vi "Ejercicio 2.3.vi"() -> ()   [LabVIEW 2021]
uses:
  <vilib>/express/express arith-compare/Formula/XNode/ExpressFormulaBlockNode.xnode
panel:
  out "Numeric 3":dbl
  in  "Numeric":dbl
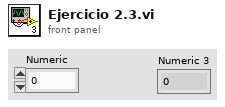
[diagram p1: front panel]
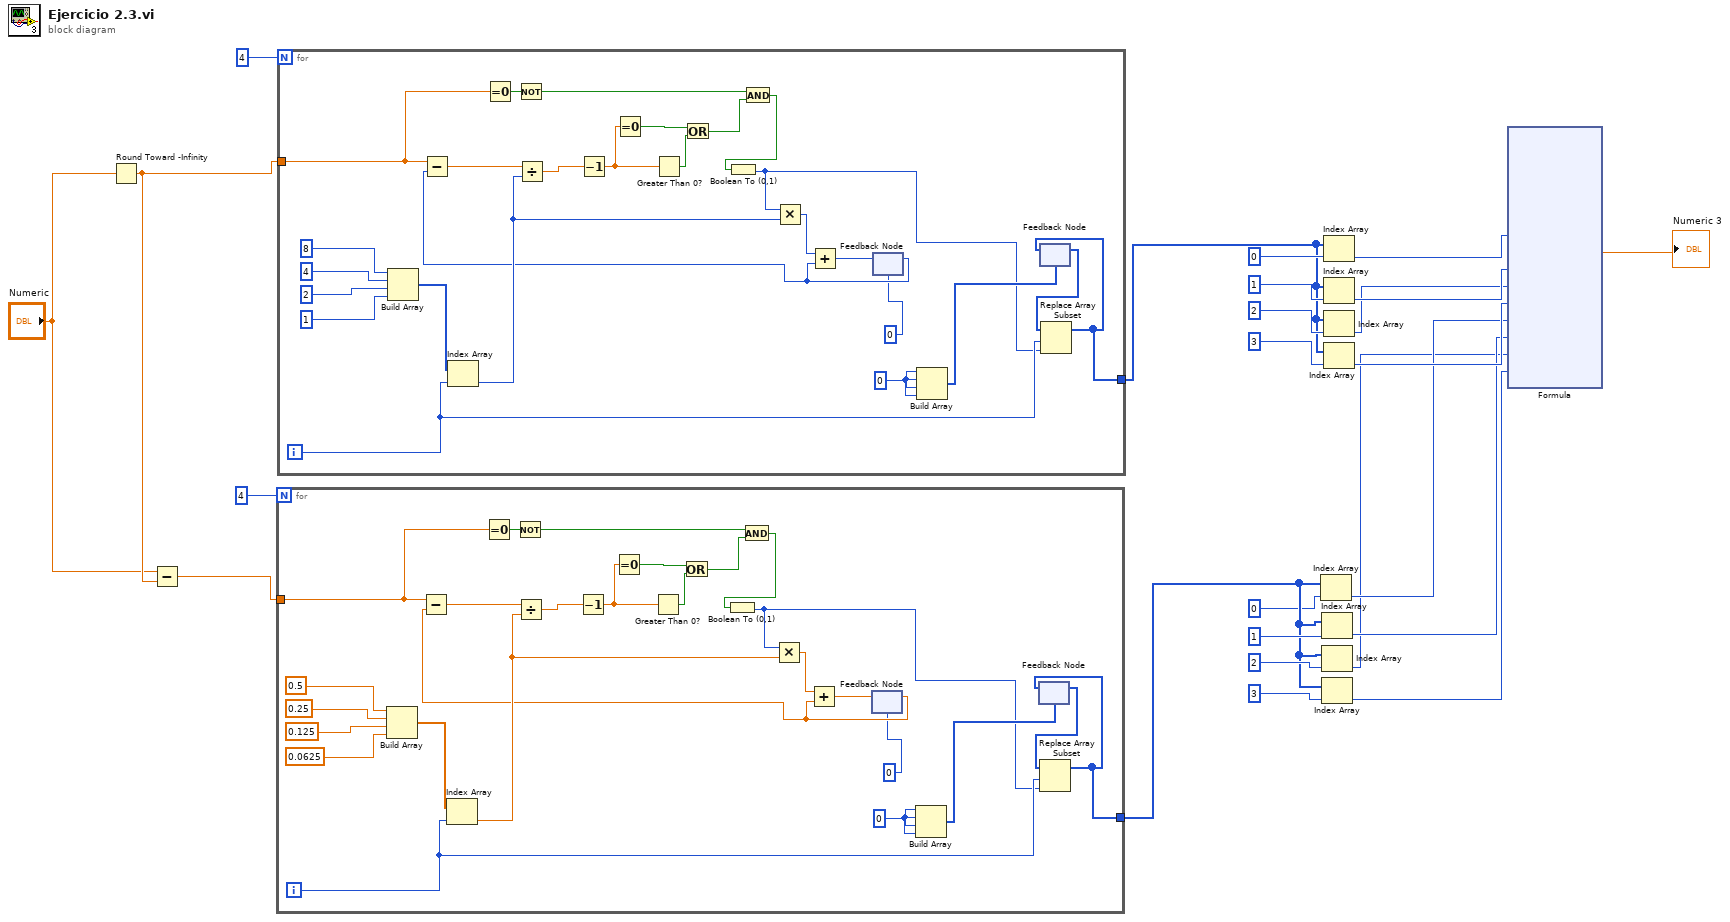
[diagram p0: block diagram]
diagram:
  n1 = Round Toward -Infinity(1:"Numeric") -> (0:w23:dbl)
  n2 = Subtract(x="Numeric", y=w23) -> (x-y=w3:dbl)
  n3 = for {
    N: 4 -> [_]
    tunnel: w3 -> [w43]
    tunnel: [w29] -> w2
    i -> [w34]
    w33 = 0
    n4 = Build Array(0.5, 0.25, 0.125, 0.0625) -> (w50:dbl[])
    n5 = Index Array(array=w50, index=w34) -> (element=w38:dbl)
    n6 = Equal To 0?(x=w43) -> (x = 0?=w45:bool)
    n7 = Not(x=w45) -> (.not. x?=w44:bool)
    n8 = feedback #1(0) -> (w36:dbl)
    n9 = Subtract(x=w43, y=w36) -> (x-y=w42:dbl)
    n10 = Divide(x=w42, y=w38) -> (x/y=w40:dbl)
    n11 = Decrement(x=w40) -> (x-1=w39:dbl)
    n12 = Equal To 0?(x=w39) -> (x = 0?=w49:bool)
    n13 = Greater Than 0?(x=w39) -> (x > 0?=w48:bool)
    n14 = Or(x=w49, y=w48) -> (x .or. y?=w46:bool)
    n15 = And(x=w44, y=w46) -> (x .and. y?=w41:bool)
    n16 = Boolean To (0,1)(Boolean=w41) -> (0, 1=w30:i16)
    n17 = Multiply(x=w30, y=w38) -> (x*y=w47:dbl)
    n18 = Add(x=w47, y=w36) -> (x+y=w37:dbl)
    n19 = feedback-in #1(w37) -> ()
    n20 = Build Array(w33, w33, w33, w33) -> (w31:i32[])
    n21 = feedback #2(w31) -> (w32:i32[])
    n22 = Replace Array Subset(array=w32, new element=w30, index=w34) -> (w29:i32[])
    n23 = feedback-in #2(w29) -> ()
  }
  n24 = for {
    N: 4 -> [_]
    tunnel: w23 -> [w65]
    tunnel: [w51] -> w17
    i -> [w56]
    w55 = 0
    n25 = Build Array(8, 4, 2, 1) -> (w72:i32[])
    n26 = Index Array(array=w72, index=w56) -> (element=w60:i32)
    n27 = Equal To 0?(x=w65) -> (x = 0?=w67:bool)
    n28 = Not(x=w67) -> (.not. x?=w66:bool)
    n29 = feedback #3(0) -> (w58:i32)
    n30 = Subtract(x=w65, y=w58) -> (x-y=w64:dbl)
    n31 = Divide(x=w64, y=w60) -> (x/y=w62:dbl)
    n32 = Decrement(x=w62) -> (x-1=w61:dbl)
    n33 = Equal To 0?(x=w61) -> (x = 0?=w71:bool)
    n34 = Greater Than 0?(x=w61) -> (x > 0?=w70:bool)
    n35 = Or(x=w71, y=w70) -> (x .or. y?=w68:bool)
    n36 = And(x=w66, y=w68) -> (x .and. y?=w63:bool)
    n37 = Boolean To (0,1)(Boolean=w63) -> (0, 1=w52:i16)
    n38 = Multiply(x=w52, y=w60) -> (x*y=w69:i32)
    n39 = Add(x=w69, y=w58) -> (x+y=w59:i32)
    n40 = feedback-in #3(w59) -> ()
    n41 = Build Array(w55, w55, w55, w55) -> (w53:i32[])
    n42 = feedback #4(w53) -> (w54:i32[])
    n43 = Replace Array Subset(array=w54, new element=w52, index=w56) -> (w51:i32[])
    n44 = feedback-in #4(w51) -> ()
  }
  n45 = Index Array(array=w2, index=0) -> (element=w9:i32)
  n46 = Index Array(array=w2, index=1) -> (element=w8:i32)
  n47 = Index Array(array=w2, index=2) -> (element=w5:i32)
  n48 = Index Array(array=w2, index=3) -> (element=w7:i32)
  n49 = Index Array(array=w17, index=0) -> (element=w11:i32)
  n50 = Index Array(array=w17, index=1) -> (element=w13:i32)
  n51 = Index Array(array=w17, index=2) -> (element=w12:i32)
  n52 = Index Array(array=w17, index=3) -> (element=w10:i32)
  n53 = xnode "Formula"("X1"=w11, "X2"=w13, "X3"=w12, "X4"=w10, "X5"=w9, "X6"=w8, "X7"=w5, "X8"=w7) -> ("Result"=→"Numeric 3":dbl)  [unwired: 1 in, 1 out]
